vi "AttrSet.vi"   [LabVIEW 2011, in "Konvolucio MCAN120803.lvlib"]
uses:
  <instrlib>/Konvolucio MCAN120803/Konvolucio MCAN120803.lvlib
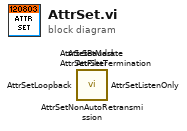
[diagram p0: block diagram]
diagram:
  n1 = call <instrlib>:"AttrSetNonAutoRetransmission.vi"() -> ()  [unwired: 9 in, 2 out]
  n2 = call <instrlib>:"AttrSetTermination.vi"() -> ()  [unwired: 9 in, 2 out]
  n3 = call <instrlib>:"AttrSetLoopback.vi"() -> ()  [unwired: 9 in, 2 out]
  n4 = call <instrlib>:"AttrSetListenOnly.vi"() -> ()  [unwired: 9 in, 2 out]
  n5 = call <instrlib>:"AttrSetMask.vi"() -> ()  [unwired: 9 in, 2 out]
  n6 = call <instrlib>:"AttrSetFilter.vi"() -> ()  [unwired: 9 in, 2 out]
  n7 = call <instrlib>:"AttrSetBaudrate.vi"() -> ()  [unwired: 9 in, 2 out]
